vi "template.vi"() -> ()   [LabVIEW 2015, in "lv-build-interface.lvlib"]
uses:
  lv-build-interface.lvlib
  lv-builder/lv-builder.lvclass
panel:
  out "results":T1(array[cluster])
  out "error":errorcluster
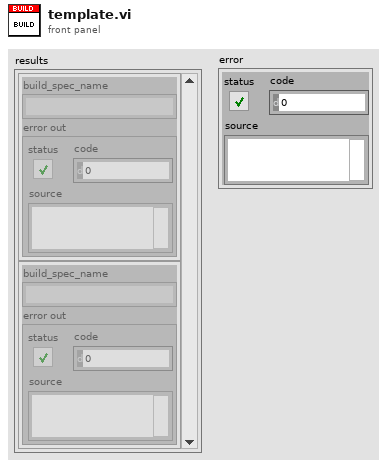
[diagram p1: front panel]
types:
  T1 = cluster{"build_spec_name":string, "error out":errorcluster}[]
  T2 = typedef "lv-build.lvlib/build_specification.ctl" = cluster{"type":T3, "build_spec_name":string, "target_name":string, "owner_name []":string[], "project_path":path, "build_destination":path, "build_artifact":path, "post_artifact":path}
  T3 = typedef "lv-build.lvlib/build_type.ctl" = enum16{"<build_type>", "application_pc", "application_rt", "installer", "llb", "lvlibp", "zip", "fpga", "<null>"}
  T4 = cluster{"build_spec_name":string, "error out":errorcluster}
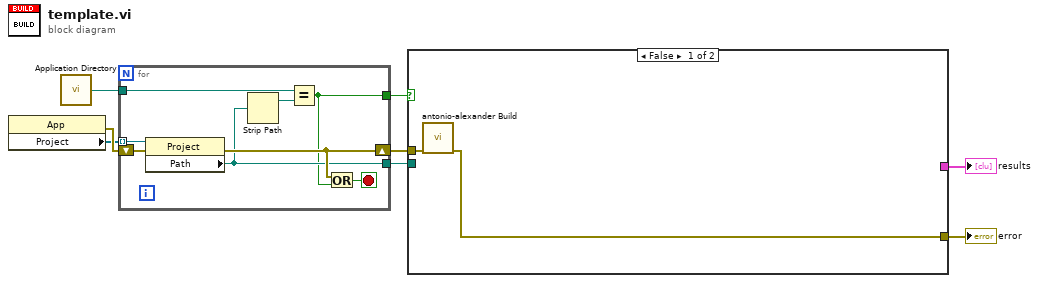
[diagram p0: block diagram]
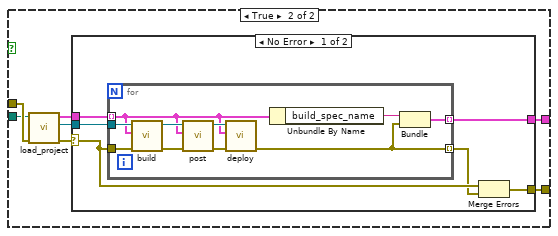
[diagram p2: hidden frame]
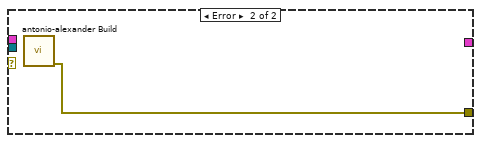
[diagram p3: hidden frame]
diagram:
  n1 = property class="App"() -> (error out=w7:errorcluster, "Project"=w6:refnum<vi>[])  [unwired: 2 in, 1 out]
  n2 = call <vilib>:"Application Directory.vi"() -> ("Application Directory"=w5:path)
  n3 = for {
    tunnel: w6 -> [w15] mode=indexing
    tunnel: w5 -> [w13]
    tunnel: [w12] -> w4
    tunnel: [w11] -> w2
    shift-right: [w16] -> w8
    shift-left: w7 -> [w10]
    stop <- w9 stop-if-true
    n4 = property class="Project"(reference=w15, error in=w10) -> (error out=w16:errorcluster, "Path"=w12:path)  [unwired: 1 out]
    n5 = Strip Path(path=w12) -> (stripped path=w14:path)  [unwired: 1 out]
    n6 = Equal?(x=w13, y=w14) -> (x = y?=w11:bool)
    n7 = Or(x=w16, y=w11) -> (x .or. y?=w9:bool)
  }
  n8 = case shown="False" w2 {
    tunnel: w8 -> [w18 w25]
    tunnel: w4 -> [_ w24]
    tunnel: [w17 w20] -> w3
    tunnel: [_ w19] -> w1
    frame False {
      n9 = call "antonio-alexander Build.vi"("error in (no error)"=w18) -> ("error out"=w17:errorcluster)  [unwired: 10 in]
    }
    frame True {
      n10 = call "load_project.vi"("error in (no error)"=w25, "project_file"=w24) -> ("error out"=w22:errorcluster, "lv-builder out"=w23:refnum<class "lv-builder.lvclass">, "build_spec_info []"=w21:T2[])  [unwired: 6 in, 1 out]
      n11 = case shown="No Error" w22 {
        selector: w22 -> [w30 _]
        tunnel: w23 -> [w31 _]
        tunnel: w21 -> [w29 _]
        tunnel: [w27 w42] -> w20
        tunnel: [w26 _] -> w19
        frame No Error {
          n12 = for {
            tunnel: w31 -> [w41]
            tunnel: w30 -> [w38]
            tunnel: [w33] -> w28 mode=indexing
            tunnel: w29 -> [w35] mode=indexing
            tunnel: [w32] -> w26 mode=indexing
            n13 = call-dynamic "build.vi"("error in (no error)"=w38, "build_spec"=w35, "lv-build-default in"=w41) -> ("error out"=w37:errorcluster, "lv-build-default out"=w40:refnum<class "lv-builder.lvclass">)  [unwired: 6 in, 1 out]
            n14 = call-dynamic "post.vi"("error in (no error)"=w37, "build_spec"=w35, "lv-build-default in"=w40) -> ("error out"=w36:errorcluster, "lv-build-default out"=w39:refnum<class "lv-builder.lvclass">)  [unwired: 7 in]
            n15 = call-dynamic "deploy.vi"("error in (no error)"=w36, "build_spec"=w35, "lv-builder in"=w39) -> ("error out"=w33:errorcluster)  [unwired: 7 in, 1 out]
            n16 = Unbundle By Name(w35) -> ("build_spec_name"=w34:string)
            n17 = Bundle("build_spec_name"=w34, "error out"=w33) -> (w32:T4)  [unwired: 1 in]
          }
          n18 = Merge Errors(w30, w28) -> (w27:errorcluster)
        }
        frame Error {
          n19 = call "antonio-alexander Build.vi"() -> ("error out"=w42:errorcluster)  [unwired: 11 in]
        }
      }
    }
  }
  "error" <- w3
  "results" <- w1
